vi "read lockin status.vi"(7 "Device channel name":string, 8 "error in (no error)":errorcluster, 11 "SRS830 address":refnum<visa-resource-name>) -> (0 "error out":errorcluster, 2 "concatenated string":string, 3 "SRS830 address 2":refnum<visa-resource-name>)   [LabVIEW 2024]
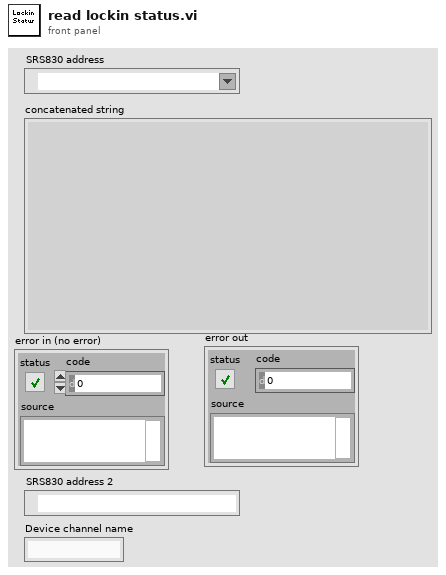
[diagram p1: front panel]
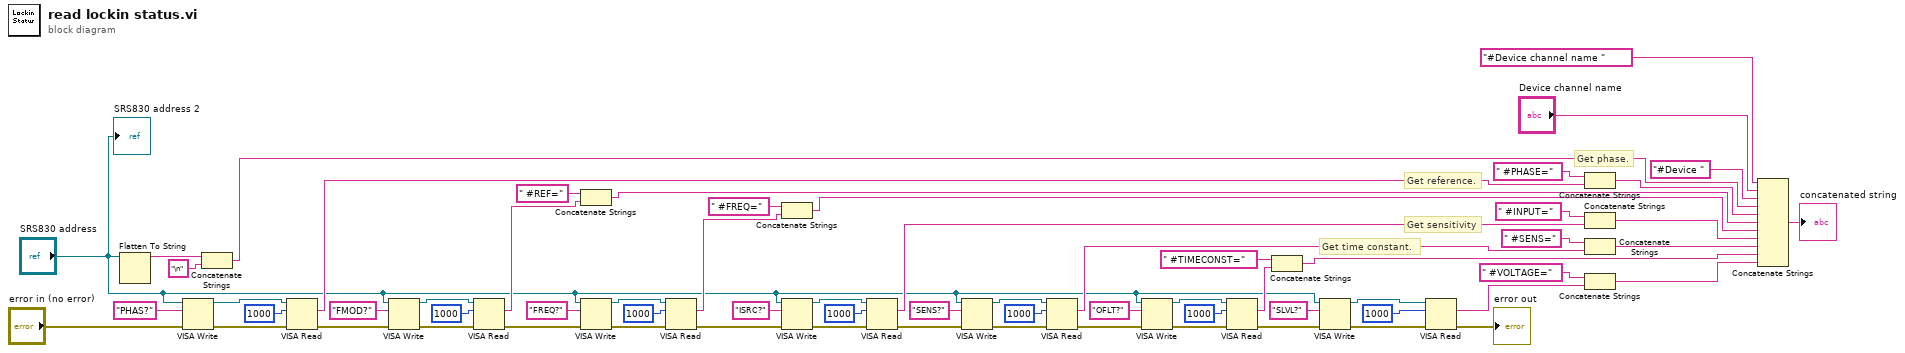
[diagram p0: block diagram]
diagram:
  # "Get time constant."
  # "Get sensitivity"
  # "Get reference."
  # "Get phase."
  n1 = Flatten To String(anything="SRS830 address") -> (data string=w5:string)  [unwired: 3 in, 2 out]
  n2 = VISA Write(VISA resource name="SRS830 address", write buffer="PHAS?", error in (no error)="error in (no error)") -> (VISA resource name out=w54:refnum<visa-resource-name>, error out=w55:errorcluster)  [unwired: 1 out]
  n3 = Concatenate Strings(w5, "\n" ("string")) -> (w4:string)
  n4 = VISA Read(VISA resource name=w54, byte count=u32 1000, error in (no error)=w55) -> (read buffer=w50:string, error out=w62:errorcluster)  [unwired: 2 out]
  n5 = VISA Write(VISA resource name="SRS830 address", write buffer="FMOD?", error in (no error)=w62) -> (VISA resource name out=w48:refnum<visa-resource-name>, error out=w49:errorcluster)  [unwired: 1 out]
  n6 = VISA Read(VISA resource name=w48, byte count=u32 1000, error in (no error)=w49) -> (read buffer=w44:string, error out=w13:errorcluster)  [unwired: 2 out]
  n7 = Concatenate Strings(" #REF=" ("string"), w44) -> (w60:string)
  n8 = VISA Write(VISA resource name="SRS830 address", write buffer="FREQ?", error in (no error)=w13) -> (VISA resource name out=w42:refnum<visa-resource-name>, error out=w43:errorcluster)  [unwired: 1 out]
  n9 = VISA Read(VISA resource name=w42, byte count=u32 1000, error in (no error)=w43) -> (read buffer=w38:string, error out=w12:errorcluster)  [unwired: 2 out]
  n10 = Concatenate Strings(" #FREQ=" ("string"), w38) -> (w59:string)
  n11 = VISA Write(VISA resource name="SRS830 address", write buffer="ISRC?", error in (no error)=w12) -> (VISA resource name out=w36:refnum<visa-resource-name>, error out=w37:errorcluster)  [unwired: 1 out]
  n12 = VISA Read(VISA resource name=w36, byte count=u32 1000, error in (no error)=w37) -> (read buffer=w32:string, error out=w11:errorcluster)  [unwired: 2 out]
  n13 = VISA Write(VISA resource name="SRS830 address", write buffer="SENS?", error in (no error)=w11) -> (VISA resource name out=w30:refnum<visa-resource-name>, error out=w31:errorcluster)  [unwired: 1 out]
  n14 = VISA Read(VISA resource name=w30, byte count=u32 1000, error in (no error)=w31) -> (read buffer=w26:string, error out=w10:errorcluster)  [unwired: 2 out]
  n15 = VISA Write(VISA resource name="SRS830 address", write buffer="OFLT?", error in (no error)=w10) -> (VISA resource name out=w24:refnum<visa-resource-name>, error out=w25:errorcluster)  [unwired: 1 out]
  n16 = VISA Read(VISA resource name=w24, byte count=u32 1000, error in (no error)=w25) -> (read buffer=w20:string, error out=w9:errorcluster)  [unwired: 2 out]
  n17 = Concatenate Strings(" #TIMECONST=" ("string"), w20) -> (w56:string)
  n18 = VISA Write(VISA resource name="SRS830 address", write buffer="SLVL?", error in (no error)=w9) -> (VISA resource name out=w18:refnum<visa-resource-name>, error out=w19:errorcluster)  [unwired: 1 out]
  n19 = VISA Read(VISA resource name=w18, byte count=u32 1000, error in (no error)=w19) -> (read buffer=w14:string, error out=→"error out":errorcluster)  [unwired: 2 out]
  n20 = Concatenate Strings(" #PHASE=" ("string"), w50) -> (w61:string)
  n21 = Concatenate Strings(" #INPUT=" ("string"), w32) -> (w58:string)
  n22 = Concatenate Strings(" #SENS=" ("string"), w26) -> (w57:string)
  n23 = Concatenate Strings(" #VOLTAGE=" ("string"), w14) -> (w65:string)
  n24 = Concatenate Strings("#Device channel name " ("string"), "Device channel name", "#Device " ("string"), w4, w61, w60, w59, w58, w57, w56, w65) -> (→"concatenated string":string)
  "SRS830 address 2" <- "SRS830 address"
